vi "Test Extra Pins.vi"() -> ()   [LabVIEW 2013]
uses:
  <vilib>/Platform/TimedLoop/XDataNode/timing_clust.ctl
  <vilib>/Platform/TimedLoop/XDataNode/nitl_modes.ctl
  <vilib>/Platform/TimedLoop/XDataNode/wakeup.ctl
  <vilib>/FPGAPlugInAG/PXI-7833R/niLvFpga_Open_PXI-7833R.vi
  <vilib>/Utility/error.llb/Error Cluster From Error Code.vi
  <vilib>/rvi/errors/niLvFpgaAdjustHostInterfaceError.vi
  <vilib>/FPGAPlugInAG/PXI-7833R/niLvFpga_Reset_PXI-7833R.vi
  <vilib>/FPGAPlugInAG/PXI-7833R/niLvFpga_Close_PXI-7833R.vi
  <vilib>/platform/TimedLoop/XDataNode/XDataNode.xnode
  <vilib>/rvi/interface/nirviOpenFPGA/nirviOpenFPGA.xnode
  FPGA Bitfiles/IRISSControl_FPGATarget_IRISSFPGAIOv3.3b_EdPqLwYMJEE.lvbitx
  IRISS_FPGA_IO_v3.3b.vi
  <vilib>/rvi/interface/nirviReadWriteControl/nirviReadWriteControl.xnode
  <vilib>/rvi/interface/nirviMethod/nirviMethod.xnode
  <vilib>/rvi/interface/nirviCloseFPGA/nirviCloseFPGA.xnode
  <vilib>/Platform/TimedLoop/XDataNode/XDNodeRunTimeDep.lvlib
  NiFpgaLv.dll
panel:
  in  "direction":bool
  in  "delay [ms]":dbl
  out "error out":errorcluster
  in  "stop":bool
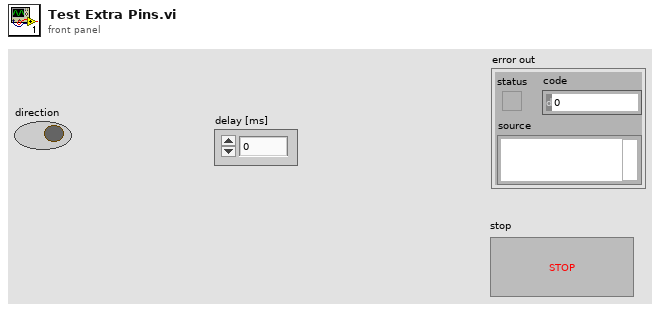
[diagram p1: front panel]
types:
  T1 = typedef "XDNodeRunTimeDep.lvlib/timing_clust.ctl" = cluster{"Expected End [f-1]":u64, "Actual End [f-1]":u64, "Finished Late? [f-1]":bool, "Expected End [i-1]":u64, "Actual End [i-1]":u64, "Finished Late? [i-1]":bool, "Expected Start [i]":u64, "Actual Start [i]":u64, "Expected Start [f]":u64, "Actual Start [f]":u64, "Source Name":string, "Structure Name":string, "Period":i64, "Deadline":i64, "Offset":i64, "Start":i64, "Priority":i32, "Timeout":i32, "Mode":T2, "Wakeup Reason":T3, "Error":errorcluster, "Source Type":string, "Secondary Source Type":string, "Global End Time":u64, "Global Start Time":u64, "Frame Duration":u64, "Iteration Duration":u64, "Assigned CPU":i32, "I/O Scan Engine Mode":u32}
  T2 = typedef "XDNodeRunTimeDep.lvlib/nitl_modes.ctl" = enum32{"No Change", "Process missed periods, maintain original phase", "Discard missed periods, maintain original phase", "Process missed periods, ignore original phase", "Discard missed periods, ignore original phase"}
  T3 = typedef "XDNodeRunTimeDep.lvlib/wakeup.ctl" = enum32{"Normal", "Aborted", "Asynchronous wakeup", "Timing source error", "Timed loop error", "Timeout"}
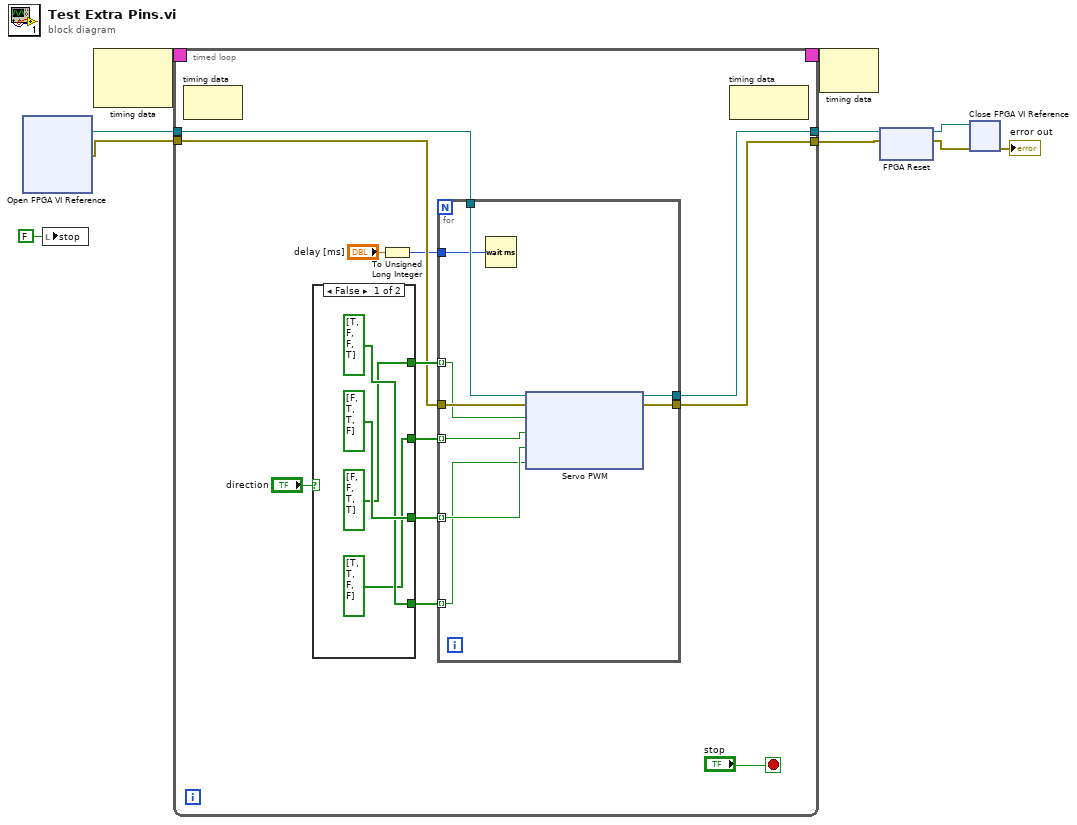
[diagram p0: block diagram]
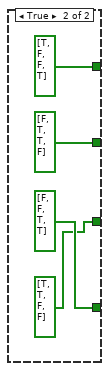
[diagram p2: hidden frame]
diagram:
  n1 = xnode "Open FPGA VI Reference"() -> ("FPGA VI Reference Out"=w8:refnum<k20>, "error out"=w7:errorcluster)  [unwired: 2 in]
  n2 = local write "stop"(FALSE ("stop")) -> ()
  n3 = node-c288() -> (w10:T1)  [unwired: 2 in]
  n4 = timed-loop {
    timing: w10 -> [_]
    timing-out: [_] -> w9
    tunnel: w8 -> [w16]
    tunnel: w7 -> [w14]
    tunnel: [w15] -> w4
    tunnel: [w13] -> w2
    stop <- "stop" stop-if-true
    n5 = node-c288() -> ()  [unwired: 1 in, 1 out]
    n6 = case shown="False" "direction" {
      tunnel: [bool[] [FALSE, FALSE, TRUE, TRUE] bool[] [TRUE, FALSE, FALSE, TRUE]] -> w21
      tunnel: [bool[] [TRUE, TRUE, FALSE, FALSE] bool[] [FALSE, TRUE, TRUE, FALSE]] -> w20
      tunnel: [bool[] [FALSE, TRUE, TRUE, FALSE] bool[] [TRUE, TRUE, FALSE, FALSE]] -> w19
      tunnel: [bool[] [TRUE, FALSE, FALSE, TRUE] bool[] [FALSE, FALSE, TRUE, TRUE]] -> w18
      frame False {
      }
      frame True {
      }
    }
    n7 = To Unsigned Long Integer(number="delay [ms]") -> (unsigned 32bit integer=w12:u32)
    n8 = for {
      tunnel: w21 -> [w35] mode=indexing
      tunnel: w20 -> [w34] mode=indexing
      tunnel: w19 -> [w33] mode=indexing
      tunnel: w18 -> [w32] mode=indexing
      tunnel: w16 -> [w39]
      tunnel: [w38] -> w15
      tunnel: w14 -> [w37]
      tunnel: [w36] -> w13
      tunnel: w12 -> [w31]
      n9 = Wait (ms)(milliseconds to wait=w31) -> ()  [unwired: 1 out]
      n10 = xnode "Servo PWM"("FPGA VI Reference In"=w39, "error in"=w37, "Connector2/DIO7"=w35, "Connector2/DIO8"=w34, "Connector2/DIO9"=w33, "Connector2/DIO10"=w32) -> ("FPGA VI Reference Out"=w38:refnum<k20>, "error out"=w36:errorcluster)
    }
    n11 = node-c288() -> ()  [unwired: 1 in, 1 out]
  }
  n12 = node-c288(w9) -> ()  [unwired: 1 out]
  n13 = xnode "FPGA Reset"("FPGA VI Reference In"=w4, "error in"=w2) -> ("FPGA VI Reference Out"=w6:refnum<k20>, "error out"=w5:errorcluster)
  n14 = xnode "Close FPGA VI Reference"("FPGA VI Reference In"=w6, "error in"=w5) -> ("error out"=→"error out":errorcluster)
